vi "Get__slk_mt.vi"(8 "error in (no error)":errorcluster, 11 "ring in":refnum<class "Ring__slk_mt.lvclass">) -> (0 "error out":errorcluster, 3 "ring out":refnum<class "Ring__slk_mt.lvclass">, 5 "value":string[](array[string]))   [LabVIEW 2012, in "Lazyboots Menu Tool.lvlib" / "Ring__slk_mt.lvclass"]
doc: "Gets the value from the control on GUI.\n\n<b>Value:</b>\n[Section, Key, Value]"
uses:
  Ring__slk_mt.lvclass
  TypeDef/TypeDef_ConnectorPattern__slk_mt.ctl
  Library/Lazyboots Menu Tool.lvlib
panel:
  # "Get__slk_mt.vi\nGets the values from the control on GUI.\n\nNOTICE -- YOU MUST LEAVE THIS NOTICE IN PLACE.\n\nCopyright (c) 2011, LIANG LIU Shawn.Liu.cn@gmail.com\nAll rights reserved.\n\nRedistribution and use in source and binary forms, with or without modification, are permitted provided that the following conditions are met:\n-Redistributions of source code must retain the above copyright notice, this list of conditions and the following disclaimer.\n-Redistributions in binary form must reproduce the above copyright notice, this list of conditions and the following disclaimer in the documentation and/or other materials provided with the distribution.\n-Neither the name of the eLp nor the names of its contributors may be used to endorse or promote products derived from this software without specific prior written permission.\n\nTHIS SOFTWARE IS PROVIDED BY THE COPYRIGHT HOLDERS AND CONTRIBUTORS \"AS IS\" AND ANY EXPRESS OR IMPLIED WARRANTIES, INCLUDING, BUT NOT LIMITED TO, THE IMPLIED WARRANTIES OF MERCHANTABILITY AND FITNESS FOR A PARTICULAR PURPOSE ARE DISCLAIMED. IN NO EVENT SHALL THE COPYRIGHT HOLDER OR CONTRIBUTORS BE LIABLE FOR ANY DIRECT, INDIRECT, INCIDENTAL, SPECIAL, EXEMPLARY, OR CONSEQUENTIAL DAMAGES (INCLUDING, BUT NOT LIMITED TO, PROCUREMENT OF SUBSTITUTE GOODS OR SERVICES; LOSS OF USE, DATA, OR PROFITS; OR BUSINESS INTERRUPTION) HOWEVER CAUSED AND ON ANY THEORY OF LIABILITY, WHETHER IN CONTRACT, STRICT LIABILITY, OR TORT (INCLUDING NEGLIGENCE OR OTHERWISE) ARISING IN ANY WAY OUT OF THE USE OF THIS SOFTWARE, EVEN IF ADVISED OF THE POSSIBILITY OF SUCH DAMAGE."
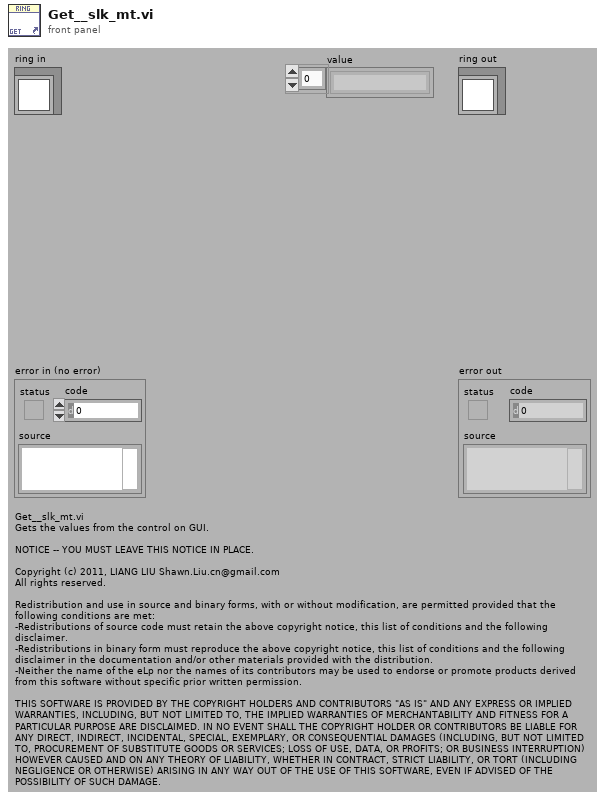
[diagram p1: front panel]
types:
  T1 = typedef "Lazyboots Menu Tool.lvlib/TypeDef_ConnectorPattern__slk_mt.ctl" = u16
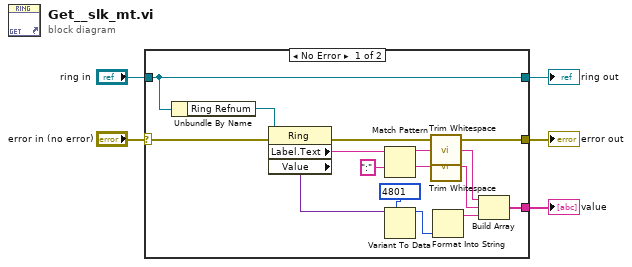
[diagram p0: block diagram]
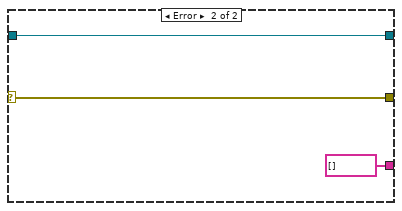
[diagram p2: hidden frame]
diagram:
  n1 = case shown="No Error" "error in (no error)" {
    selector: "error in (no error)" -> [w8 w23]
    tunnel: [w14 w23] -> w5
    tunnel: [w13 string[] []] -> w4
    tunnel: "ring in" -> [w6 w21]
    tunnel: [w6 w21] -> w1
    frame No Error {
      w12 = T1 4801 items=["4801"=4801, "4805"=4805, "4810"=4810, "4812"=4812, "4815"=4815, "4820"=4820, "4826"=4826, "4833"=4833, "4834"=4834, "4835"=4835] ("Add Error: Connector Pattern")
      n2 = Unbundle By Name(w6) -> ("Ring Refnum"=w7:refnum<vi>)
      n3 = property class="Ring"(reference=w7, error in=w8) -> (error out=w14:errorcluster, "Label.Text"=w20:string, "Value"=w11:variant)  [unwired: 1 out]
      n4 = Match Pattern(string=w20, regular expression=":") -> (before substring=w18:string, after substring=w17:string)  [unwired: 1 in, 2 out]
      n5 = Variant To Data(type=w12, Variant=w11) -> (data=w10:T1)  [unwired: 1 in, 1 out]
      n6 = call <vilib>:"Trim Whitespace.vi"("string"=w18) -> ("trimmed string"=w16:string)  [unwired: 1 in]
      n7 = call <vilib>:"Trim Whitespace.vi"("string"=w17) -> ("trimmed string"=w15:string)  [unwired: 1 in]
      n8 = Format Into String(w10) -> (resulting string=w9:string)  [unwired: 3 in, 1 out]
      n9 = Build Array(w16, w15, w9) -> (w13:string[])
    }
    frame Error {
    }
  }
  "error out" <- w5
  "ring out" <- w1
  "value" <- w4
